vi "GoPro StartStop Preview.vi"(10 "PV?":bool, 11 "Gopro DevRef":T1) -> (3 "Output DevRef":T1)   [LabVIEW 2015]
uses:
  GoPro DevRef.ctl
  <vilib>/httpClient/ClientHandle.ctl
  GET Parameter.ctl
  <vilib>/httpClient/LabVIEWHTTPClient.lvlib
panel:
  out "headers":string
  out "body":string
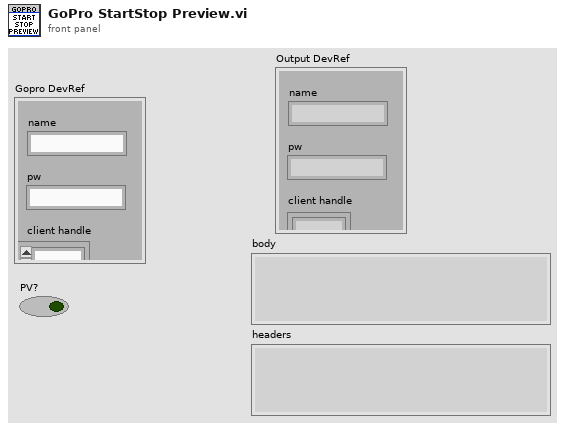
[diagram p1: front panel]
types:
  T1 = typedef "GoPro DevRef.ctl" = cluster{"name":string, "pw":string, "client handle":T2}
  T2 = typedef "LabVIEWHTTPClient.lvlib/ClientHandle.ctl" = refnum<k1>
  T3 = typedef "GET Parameter.ctl" = cluster{"key":string, "val":string}
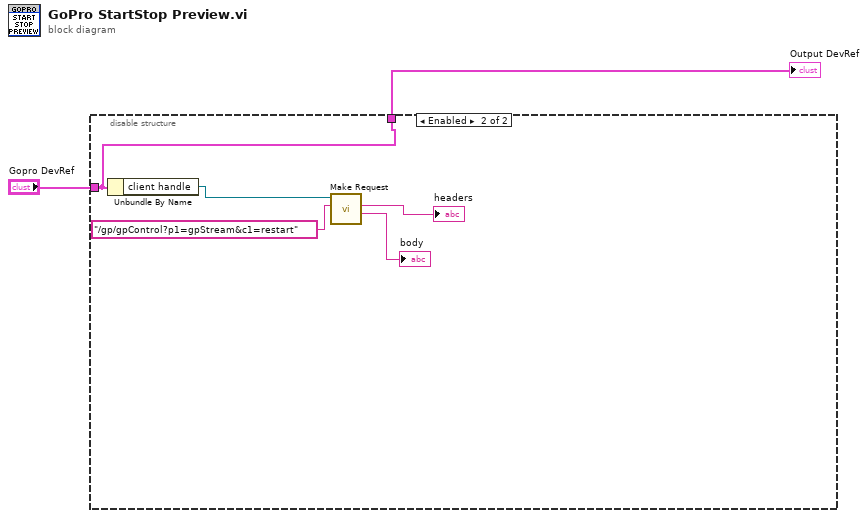
[diagram p0: block diagram]
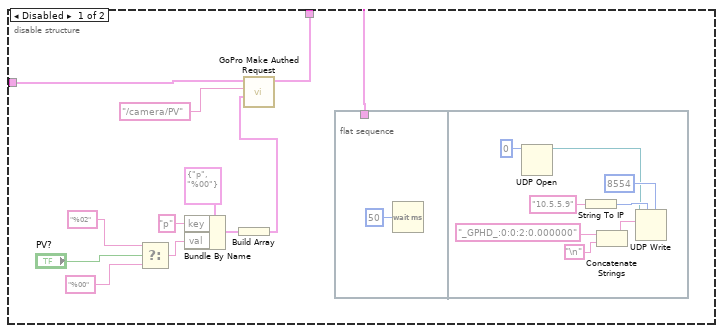
[diagram p2: hidden frame]
diagram:
  n1 = disable-structure shown="Enabled" {
    disable-tunnel: "Gopro DevRef" -> [w4 w25]
    disable-tunnel: [w3 w25] -> w1
    frame Disabled {
      n2 = Select(t="%02" ("key"), s="PV?", f="%00" ("key")) -> (s? t:f=w7:string)
      n3 = Bundle By Name(cluster=T3 {"key"="p", "val"="%00"} ("element"), "key"="p", "val"=w7) -> (w11:T3)
      n4 = Build Array(w11) -> (w12:T3[])
      n5 = call "GoPro Make Authed Request.vi"("Params"=w12, "url"="/camera/PV", "Gopro DevRef"=w4) -> ("Output DevRef"=w3:T1)  [unwired: 5 in, 3 out]
      n6 = flat-sequence {
        tunnel: w3 -> [_]
        frame #0 {
          n7 = Wait (ms)(milliseconds to wait=u32 50) -> ()  [unwired: 1 out]
        }
        frame #1 {
          n8 = UDP Open(11:u16 0 ("port")) -> (port=w16:refnum<k16>)  [unwired: 4 in, 2 out]
          n9 = String To IP(1:"10.5.5.9" ("name")) -> (0:w22:u32)
          n10 = Concatenate Strings("_GPHD_:0:0:2:0.000000" ("data in"), "\n") -> (w19:string)
          n11 = UDP Write(address=w22, port or service name=u16 8554, connection ID=w16, data in=w19) -> ()  [unwired: 2 in, 2 out]
        }
      }
    }
    frame Enabled {
      n12 = Unbundle By Name(w25) -> ("client handle"=w27:T2)
      n13 = call "Make Request.vi"("url"="/gp/gpControl?p1=gpStream&c1=restart", "Refnum in"=w27) -> ("body"=→"body":string, "headers"=→"headers":string)  [unwired: 6 in, 2 out]
    }
  }
  "Output DevRef" <- w1
